vi "setTxPower.vi"(9 "db":u16=100 max=2600, 11 "ComPort":refnum<visa-resource-name>="COM10") -> (0 "error out":errorcluster, 2 "OK":bool)   [LabVIEW 2018]
panel:
  out "read butes row":u8[](array[numeric]) format="%x"
  out "Check":u8
  # "Set TX Pover"
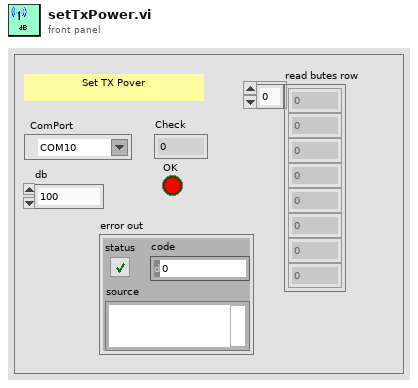
[diagram p1: front panel]
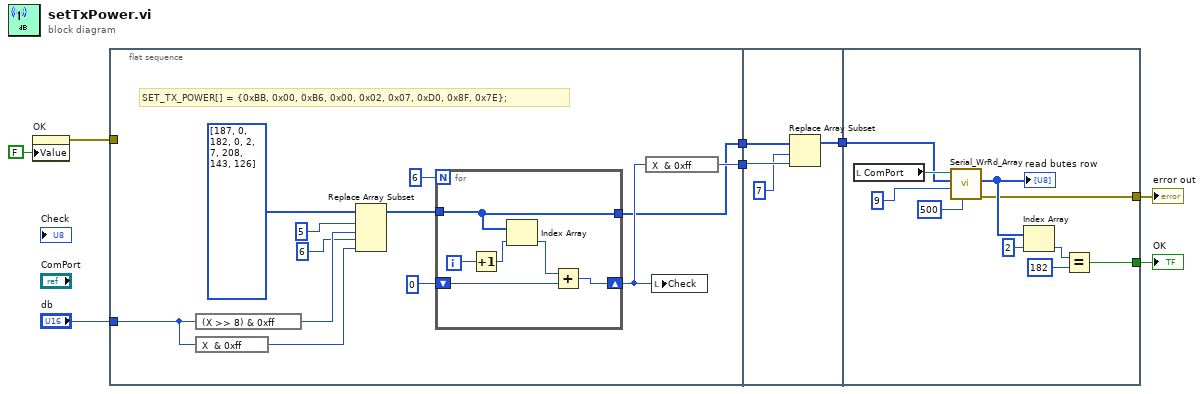
[diagram p0: block diagram]
diagram:
  n1 = property on="OK" class="Bool (strict)"("Value"=FALSE ("OK")) -> (error out=w1:errorcluster)  [unwired: 2 in, 1 out]
  n2 = flat-sequence {
    tunnel: "db" -> [w20]
    tunnel: [w9] -> w7
    tunnel: [w10] -> w6
    tunnel: w1 -> [_]
    tunnel: w7 -> [w30]
    tunnel: w6 -> [w29]
    tunnel: [w27] -> w5
    tunnel: w5 -> [w39]
    tunnel: [w32] -> w4
    tunnel: [w31] -> w3
    frame #0 {
      # "SET_TX_POWER[] = {0xBB, 0x00, 0xB6, 0x00, 0x02, 0x07, 0xD0, 0x8F, 0x7E};"
      n3 = expression code="(X >> 8) & 0xff"(w20) -> (w19:u16)
      n4 = expression code="X  & 0xff"(w20) -> (w17:u16)
      n5 = Replace Array Subset(array=u8[] [187, 0, 182, 0, 2, 7, 208, 143, 126], new element #1=w19, index #1=5 ("index"), new element #2=w17, index #2=6 ("index")) -> (w14:u8[])
      n6 = for {
        N: 6 -> [_]
        tunnel: w14 -> [w21]
        shift-right: [w24] -> w11
        shift-left: u8 0 -> [w25]
        tunnel: [w21] -> w9
        i -> [w22]
        n7 = Increment(x=w22) -> (x+1=w23:i32)
        n8 = Index Array(array=w21, index=w23) -> (element=w26:u8)
        n9 = Add(x=w26, y=w25) -> (x+y=w24:u8)
      }
      n10 = expression code="X  & 0xff"(w11) -> (w10:u8)
      n11 = local write "Check"(w11) -> ()
    }
    frame #1 {
      n12 = Replace Array Subset(array=w30, new element=w29, index=7) -> (w27:u8[])
    }
    frame #2 {
      n13 = local read "ComPort"() -> (w40:refnum<visa-resource-name>)
      n14 = call "Serial_WrRd_Array.vi"("Read Delay (ms)"=u16 500, "WR Size"=u16 9, "Array"=w39, "ComPort"=w40) -> ("error out"=w31:errorcluster, "read butes row"=w36:u8[])  [unwired: 5 in, 1 out]
      "read butes row" <- w36
      n15 = Index Array(array=w36, index=2) -> (element=w34:u8)
      n16 = Equal?(x=w34, y=u8 182) -> (x = y?=w32:bool)
    }
  }
  "OK" <- w4
  "error out" <- w3
